vi "Utility_Read_Fluid_Cluster.vi"(6 "error in (no error)":errorcluster, 9 "Fluid File":path) -> (0 "error out":errorcluster, 3 "Fluid Cluster":T1)   [LabVIEW 2016]
doc: "Reads the .mix file from the disk and retruns a cluster specifying the composition of the fluid.\n\nDeveloped by:\nGreg Sussman\nProcess Automation Corp\nwww.processauto.com\n(267)685-1249"
uses:
  Ctl/Mixture Composition cluster_d.ctl
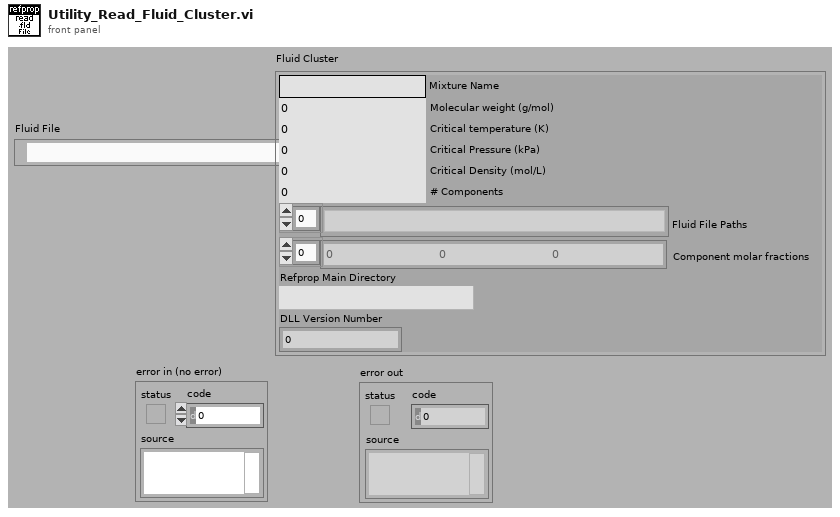
[diagram p1: front panel]
types:
  T1 = typedef "Mixture Composition cluster_d.ctl" = cluster{"Mixture Name":string, "Molecular weight (g/mol)":dbl, "Critical temperature (K)":dbl, "Critical Pressure (kPa)":dbl, "Critical Density (mol/L)":dbl, "# Components":i32, "Fluid File Paths":path[], "Component molar fractions":dbl[], "Refprop Main Directory":path, "DLL Version Number":dbl}
  T2 = enum16{"open", "open or create", "create or replace", "create", "open (read only)"}
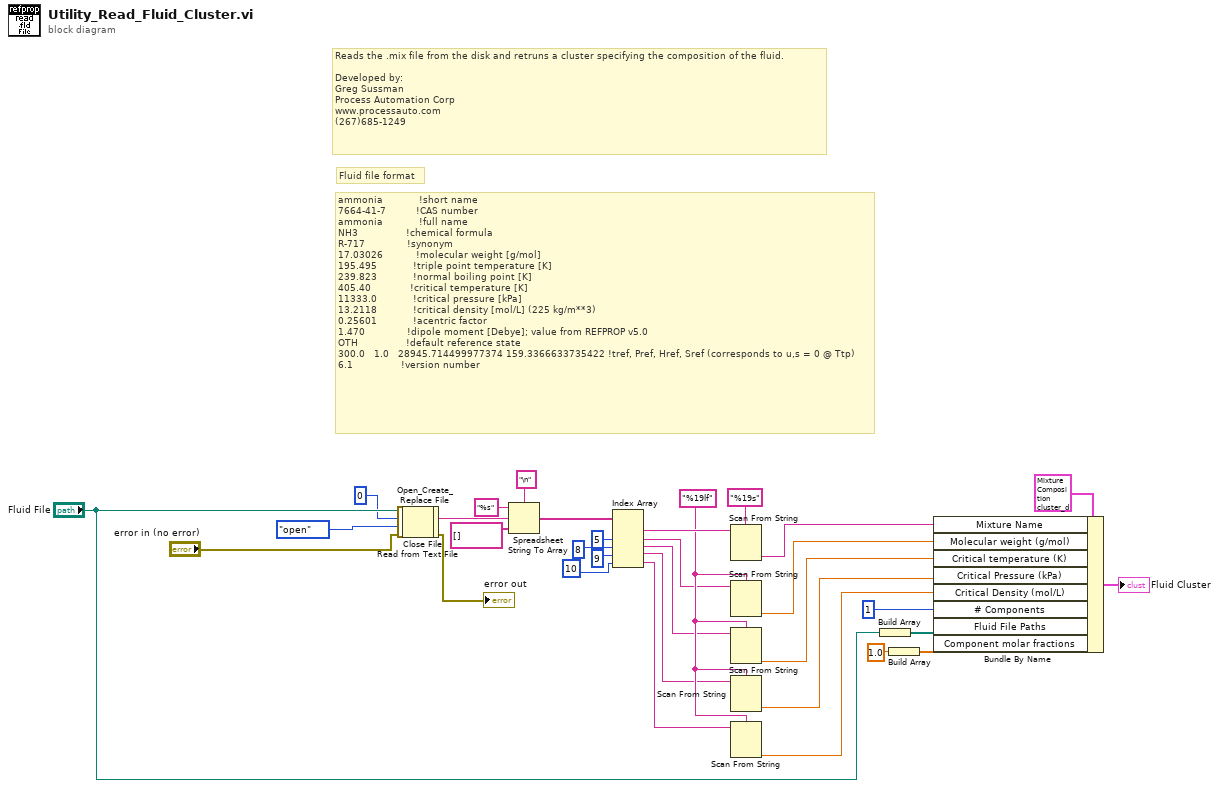
[diagram p0: block diagram]
diagram:
  w16 = "%19lf"
  # "Reads the .mix file from the disk and retruns a cluster specifying the composition of the fluid.\n\nDeveloped by:\nGreg Sussman\nProcess Automation Corp\nwww.processauto.com\n(267)685-1249"
  # "Fluid file format"
  # "ammonia            !short name\n7664-41-7          !CAS number\nammonia            !full name\nNH3                !chemical formula\nR-717              !synonym\n17.03026           !molecular weight [g/mol]\n195.495            !triple point temperature [K]\n239.823            !normal boiling point [K]\n405.40             !critical temperature [K]\n11333.0            !critical pressure [kPa]\n13.2118            !critical density [mol/L] (225 kg/m**3)\n0.25601            !acentric factor\n1.470              !dipole moment [Debye]; value from REFPROP v5.0\nOTH                !default reference state\n300.0   1.0   28945.714499977374 159.3366633735422 !tref, Pref, Href, Sref (corresponds to u,s = 0 @ Ttp)\n6.1                !version number"
  n1 = call <vilib>:"Open_Create_Replace File.vi"("error in (no error)"="error in (no error)", "function (open:0)"=T2."open", "file path"="Fluid File") -> ("error out"=w5:errorcluster, "refnum"=w4:refnum<file>)  [unwired: 5 in, 2 out]
  n2 = Read from Text File(file (use dialog)=w4, count=0 ("计数"), error in=w5) -> (refnum out=w2:refnum<file>, text=w30:string, error out=w3:errorcluster)  [unwired: 1 in, 1 out]
  n3 = Close File(refnum=w2, error in=w3) -> (error out=→"error out":errorcluster)  [unwired: 1 out]
  n4 = Spreadsheet String To Array(delimiter (Tab)="\n", format string="%s", spreadsheet string=w30, array type (2D Dbl)=string[] []) -> (array=w33:string[])
  n5 = Index Array(array=w33, index #2=5 ("index"), index #3=8 ("index"), index #4=9 ("index"), index #5=10 ("index")) -> (element #1=w18:string, element #2=w11:string, element #3=w10:string, element #4=w9:string, element #5=w8:string)  [unwired: 1 in]
  n6 = Scan From String(format string="%19s", input string=w18) -> (output 1=w17:string)  [unwired: 3 in, 3 out]
  n7 = Scan From String(format string=w16, input string=w11) -> (output 1=w15:dbl)  [unwired: 3 in, 3 out]
  n8 = Scan From String(format string=w16, input string=w10) -> (output 1=w14:dbl)  [unwired: 3 in, 3 out]
  n9 = Scan From String(format string=w16, input string=w9) -> (output 1=w13:dbl)  [unwired: 3 in, 3 out]
  n10 = Scan From String(format string=w16, input string=w8) -> (output 1=w12:dbl)  [unwired: 3 in, 3 out]
  n11 = Build Array("Fluid File") -> (w20:path[])
  n12 = Build Array(1.0) -> (w22:dbl[])
  n13 = Bundle By Name(cluster=T1 {"Mixture Name"="", "Molecular weight (g/mol)"=0.0, "Critical temperature (K)"=0.0, "Critical Pressure (kPa)"=0.0, "Critical Density (mol/L)"=0.0, "# Components"=0, "Fluid File Paths"=[], "Component molar fractions"=[], "Refprop Main Directory"=path "", "DLL Version Number"=0.0} ("Mixure Cluster"), "Mixture Name"=w17, "Molecular weight (g/mol)"=w15, "Critical temperature (K)"=w14, "Critical Pressure (kPa)"=w13, "Critical Density (mol/L)"=w12, "# Components"=1, "Fluid File Paths"=w20, "Component molar fractions"=w22) -> (→"Fluid Cluster":T1)
